vi "initializer.vi"(4 "Break":refnum<vi>) -> (0 "Cancelled?":bool, 2 "Dataflow Out":errorcluster)   [LabVIEW 2019]
panel:
  out "Button Cluster":T1
  out "Load Button Cluster":T2
  out "File Cluster":T3
  in  "Cancel Button":bool
  out "Endtime":dbl
  out "Starttime":dbl
  in  "Load Simulation File":bool
  out "Sim File Loaded":bool
  in  "LUA Simulation File":path
  out "Spec File Loaded":bool
  in  "Save Specs":bool
  out "Vali File Loaded":bool
  in  "Load Spec File":bool
  in  "Load Vali File":bool
  in  "LUA Specification File":path
  in  "LUA Validation File":path
  in  "Validate":bool
  out "# Lines":i32
  in  "Refresh Button":bool
  in  "Parameters":string(tree)="_3"
  in  "Run":bool
  # "Biogas Initializer"
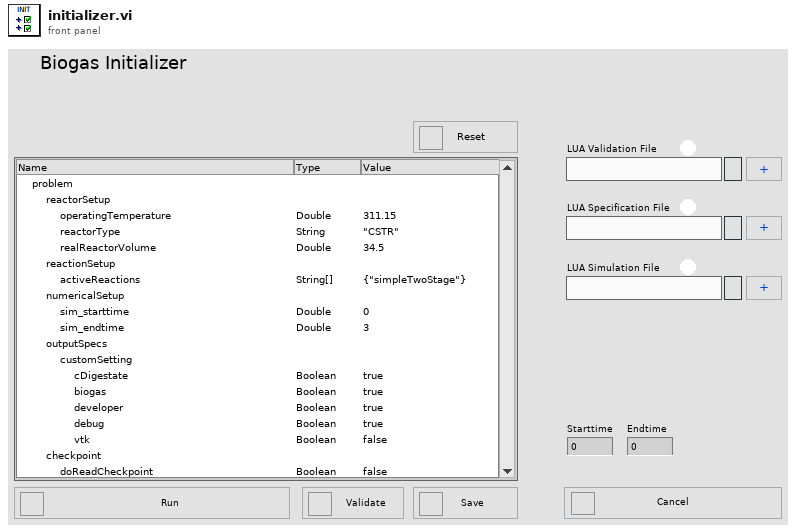
[diagram p1: front panel]
types:
  T1 = cluster{"Save Specs Button":refnum<vi>, "Cancel Button":refnum<vi>, "Run Button":refnum<vi>, "Refresh Button":refnum<vi>, "Validate Button":refnum<vi>}
  T2 = cluster{"Load Vali File":refnum<vi>, "Load Spec File":refnum<vi>, "Load Simulation File":refnum<vi>}
  T3 = cluster{"Sim File Loaded":refnum<vi>, "Vali File Loaded":refnum<vi>, "Spec File Loaded":refnum<vi>}
  T4 = cluster{"Vali File Loaded":refnum<vi>, "Spec File Loaded":refnum<vi>, "Sim File Loaded":refnum<vi>}
  T5 = typedef "LVPoint32TypeDef.ctl" = cluster{"Horizontal":i32, "Vertical":i32}
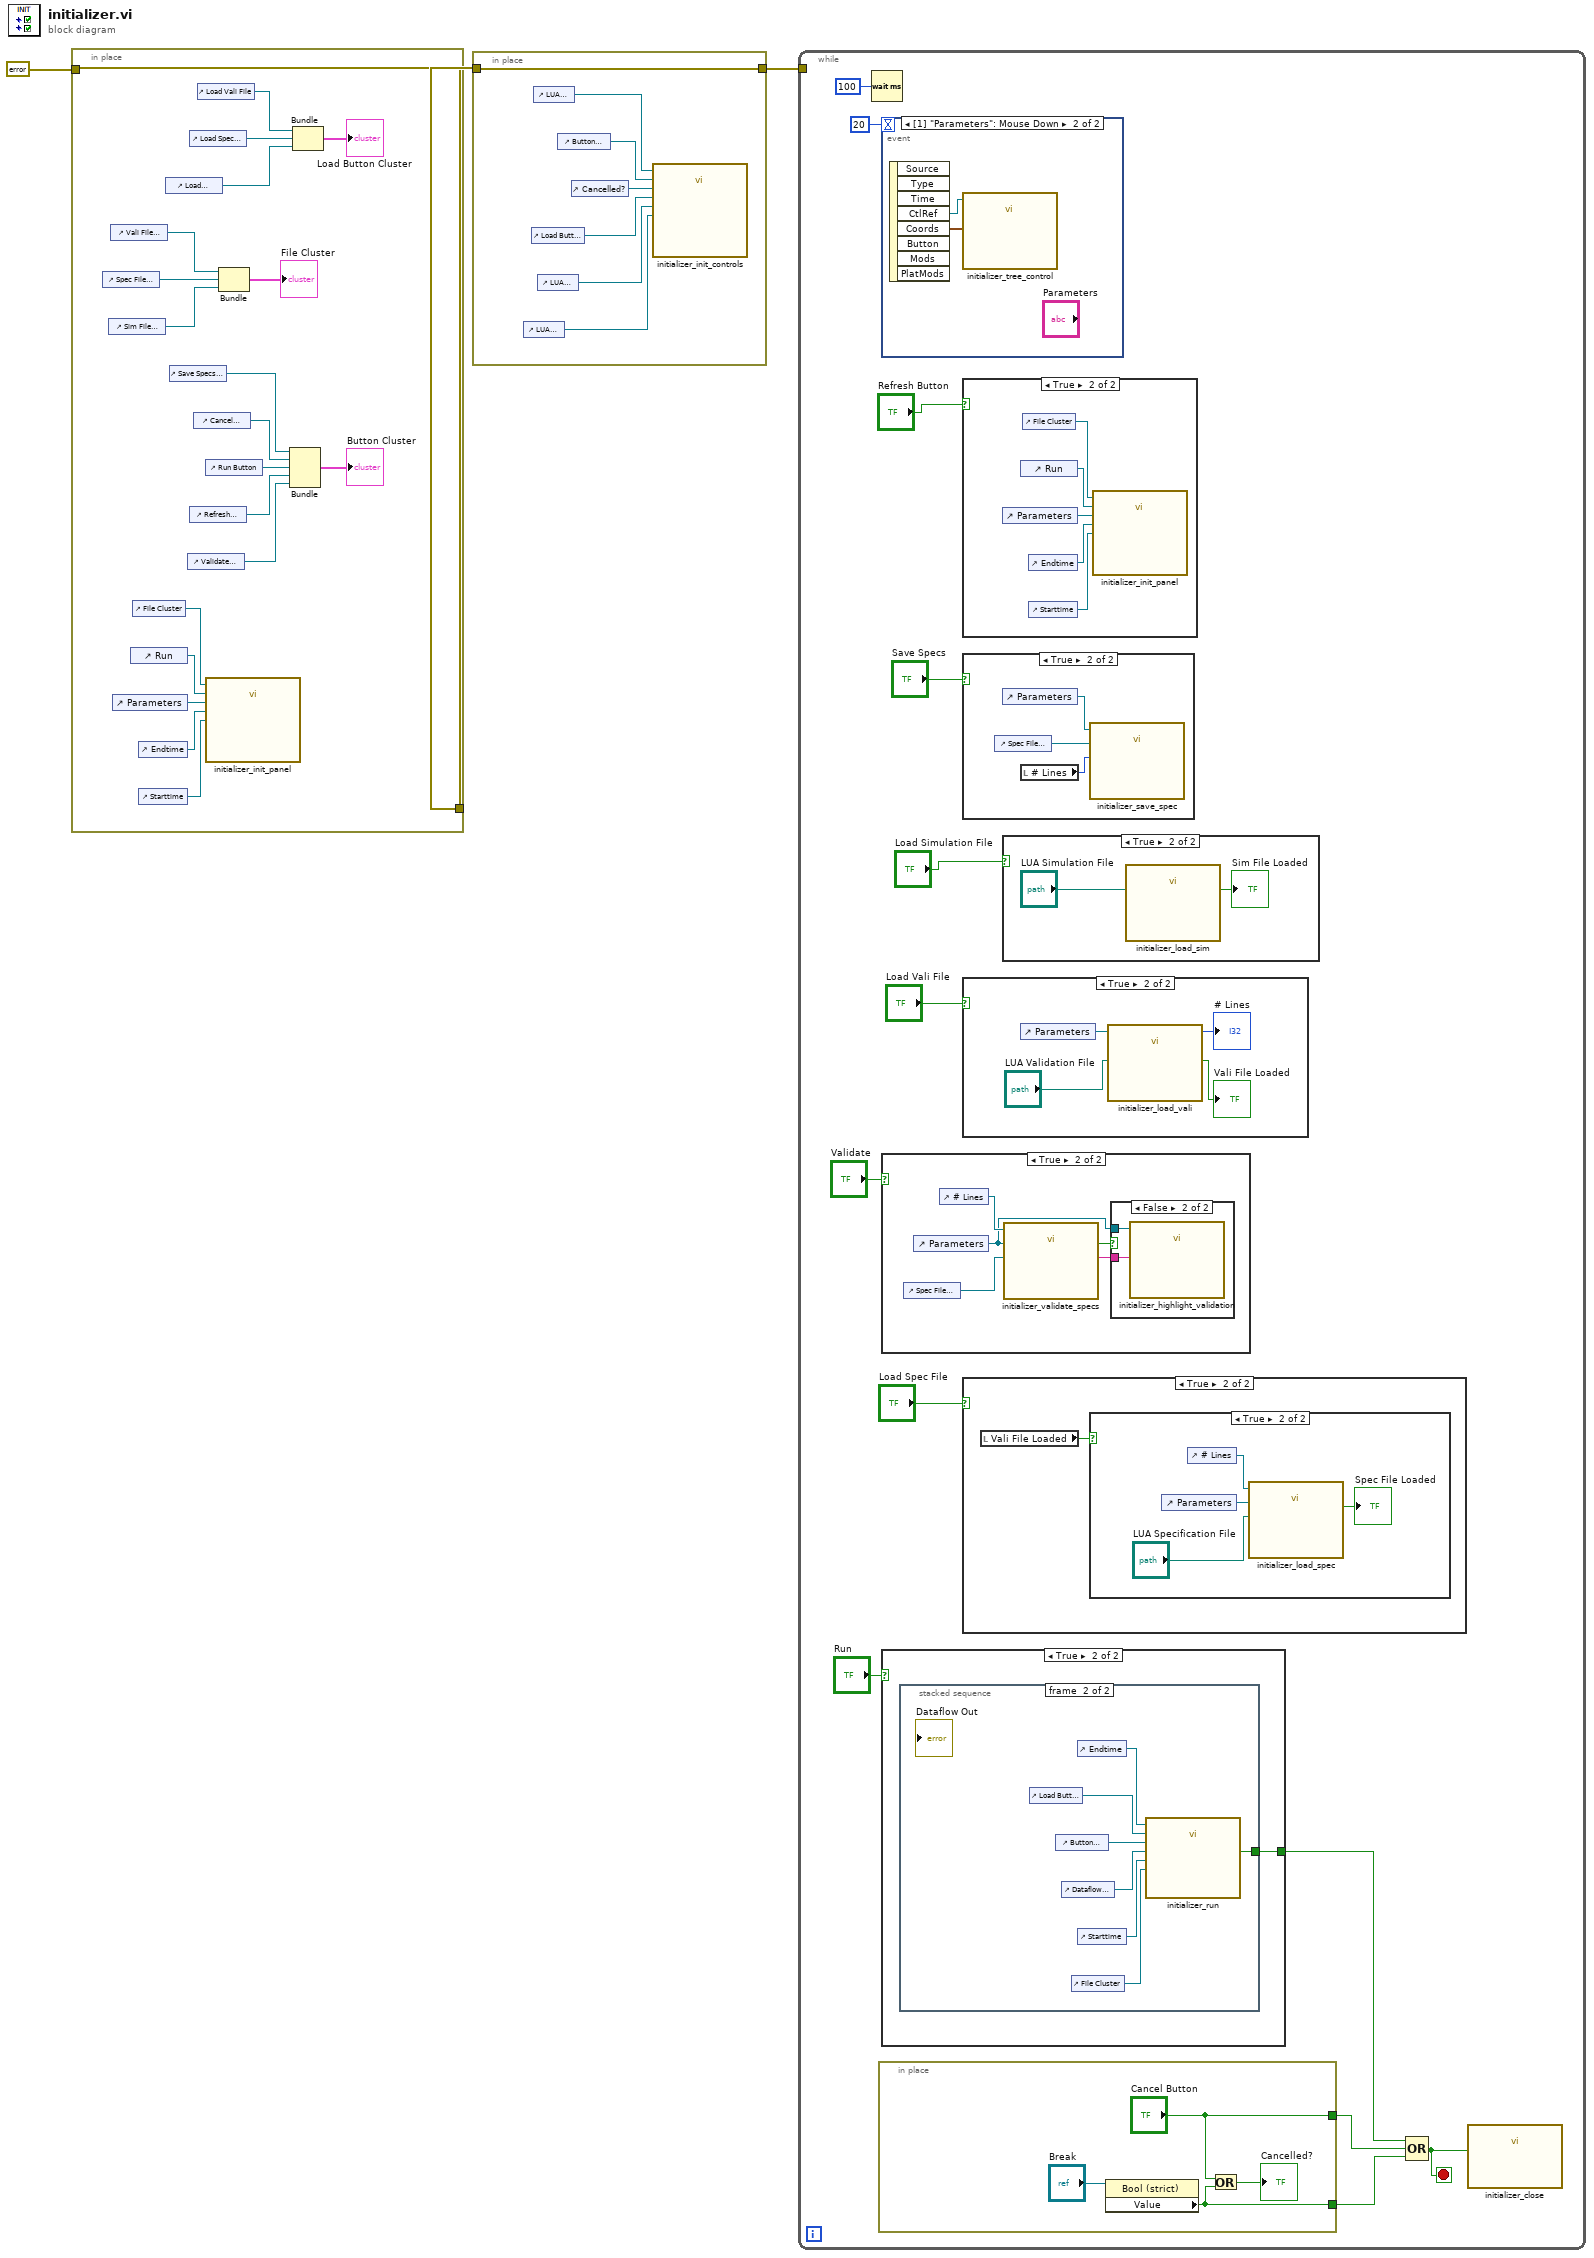
[diagram p0: block diagram]
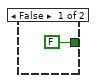
[diagram p2: hidden frame]
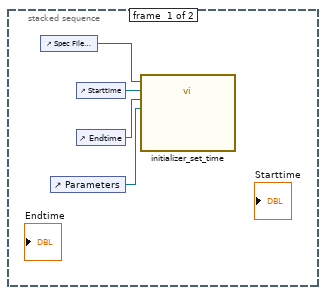
[diagram p3: hidden frame]
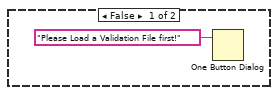
[diagram p9: hidden frame]
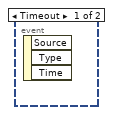
[diagram p11: hidden frame]
diagram:
  n1 = in-place {
    in-place-border: errorcluster {"status"=FALSE, "code"=0, "source"=""} ("error constant") -> [w19]
    in-place-border: [w19] -> w2
    n2 = control-ref of="Spec File Loaded"() -> (w11:refnum<vi>)
    n3 = control-ref of="Sim File Loaded"() -> (w12:refnum<vi>)
    n4 = control-ref of="Vali File Loaded"() -> (w10:refnum<vi>)
    n5 = control-ref of="Parameters"() -> (w23:refnum<vi>)
    n6 = control-ref of="Run"() -> (w20:refnum<vi>)
    n7 = control-ref of="File Cluster"() -> (w17:refnum<vi>)
    n8 = control-ref of="Endtime"() -> (w22:refnum<vi>)
    n9 = control-ref of="Starttime"() -> (w21:refnum<vi>)
    n10 = control-ref of="Load Simulation File"() -> (w14:refnum<vi>)
    n11 = control-ref of="Save Specs Button"() -> (w5:refnum<vi>)
    n12 = control-ref of="Validate Button"() -> (w9:refnum<vi>)
    n13 = control-ref of="Load Spec File"() -> (w15:refnum<vi>)
    n14 = control-ref of="Refresh Button"() -> (w8:refnum<vi>)
    n15 = control-ref of="Cancel Button"() -> (w6:refnum<vi>)
    n16 = control-ref of="Load Vali File"() -> (w16:refnum<vi>)
    n17 = control-ref of="Run Button"() -> (w7:refnum<vi>)
    n18 = call "initializer_init_panel.vi"("File Cluster"=w17, "Starttime"=w21, "Endtime"=w22, "Run Button"=w20, "Parameters Tree"=w23) -> ()  [unwired: 11 in]
    n19 = Bundle("Vali File Loaded"=w10, "Spec File Loaded"=w11, "Sim File Loaded"=w12) -> (→"File Cluster":T4)  [unwired: 1 in]
    n20 = Bundle("Save Specs Button"=w5, "Cancel Button"=w6, "Run Button"=w7, "Refresh Button"=w8, "Validate Button"=w9) -> (→"Button Cluster":T1)  [unwired: 1 in]
    n21 = Bundle("Load Vali File"=w16, "Load Spec File"=w15, "Load Simulation File"=w14) -> (→"Load Button Cluster":T2)  [unwired: 1 in]
  }
  n22 = in-place {
    in-place-border: [w30] -> w1
    in-place-border: w2 -> [w30]
    n23 = control-ref of="LUA Specification File"() -> (w27:refnum<vi>)
    n24 = control-ref of="Load Button Cluster"() -> (w25:refnum<vi>)
    n25 = control-ref of="LUA Simulation File"() -> (w28:refnum<vi>)
    n26 = control-ref of="LUA Validation File"() -> (w26:refnum<vi>)
    n27 = control-ref of="Button Cluster"() -> (w24:refnum<vi>)
    n28 = control-ref of="Cancelled?"() -> (w29:refnum<vi>)
    n29 = call "initializer_init_controls.vi"("LUA Simulation File"=w28, "Button Cluster"=w24, "Cancelled?"=w29, "Load Button Cluster"=w25, "LUA Specification File"=w27, "LUA Validation File"=w26) -> ()  [unwired: 14 in]
  }
  n30 = while {
    tunnel: w1 -> [_]
    stop <- w33 stop-if-true
    n31 = Wait (ms)(milliseconds to wait=u32 100) -> ()  [unwired: 1 out]
    n32 = in-place {
      in-place-border: ["Cancel Button"] -> w32
      in-place-border: [w44] -> w31
      n33 = property class="Bool (strict)"(reference="Break") -> ("Value"=w44:bool)  [unwired: 1 in, 2 out]
      n34 = Or(x="Cancel Button", y=w44) -> (x .or. y?=→"Cancelled?":bool)
    }
    n35 = event shown="[1] \"Parameters\": Mouse Down" {
      selector: _ -> [_ _]
      dyn-events: _ -> [_ _]
      timeout: 20 -> [_ _]
      event Timeout {
        n36 = event-data() -> ()  [unwired: 1 in, 3 out]
      }
      event "Parameters": Mouse Down {
        n37 = event-data() -> ("CtlRef"=w83:refnum<vi>, "Coords"=w84:T5)  [unwired: 1 in, 6 out]
        n38 = call "initializer_tree_control.vi"("Point"=w84, "Parameters Tree"=w83) -> ()  [unwired: 10 in]
      }
    }
    n39 = case shown="True" "Validate" {
      frame False {
      }
      frame True {
        n40 = control-ref of="Spec File Loaded"() -> (w67:refnum<vi>)
        n41 = control-ref of="Parameters"() -> (w68:refnum<vi>)
        n42 = control-ref of="# Lines"() -> (w70:refnum<vi>)
        n43 = call "initializer_validate_specs.vi"("Spec File Loaded?"=w67, "Parameters Tree"=w68, "# Lines"=w70) -> ("validationErrors"=w69:string, "Valid?"=w66:bool)  [unwired: 6 in, 1 out]
        n44 = case shown="False" w66 {
          tunnel: w69 -> [_ w72]
          tunnel: w68 -> [_ w71]
          frame True {
          }
          frame False {
            n45 = call "initializer_highlight_validation.vi"("validationErrors"=w72, "Parameters Tree"=w71) -> ()  [unwired: 10 in]
          }
        }
      }
    }
    n46 = case shown="True" "Run" {
      tunnel: [FALSE w49] -> w34
      frame False {
      }
      frame True {
        n47 = stacked-sequence {
          tunnel: [_ w60] -> w49
          frame #0 {
            n48 = control-ref of="Spec File Loaded"() -> (w51:refnum<vi>)
            n49 = control-ref of="Parameters"() -> (w50:refnum<vi>)
            n50 = control-ref of="Starttime"() -> (w53:refnum<vi>)
            n51 = control-ref of="Endtime"() -> (w52:refnum<vi>)
            n52 = call "initializer_set_time.vi"("Parameters Tree"=w50, "Endtime"=w52, "Starttime"=w53, "Spec File Loaded?"=w51) -> ()  [unwired: 8 in]
          }
          frame #1 {
            n53 = control-ref of="Load Button Cluster"() -> (w55:refnum<vi>)
            n54 = control-ref of="Button Cluster"() -> (w54:refnum<vi>)
            n55 = control-ref of="Dataflow Out"() -> (w59:refnum<vi>)
            n56 = control-ref of="File Cluster"() -> (w56:refnum<vi>)
            n57 = control-ref of="Endtime"() -> (w57:refnum<vi>)
            n58 = control-ref of="Starttime"() -> (w58:refnum<vi>)
            n59 = call "initializer_run.vi"("Endtime"=w57, "Load Button Cluster"=w55, "Button Cluster"=w54, "Dataflow Out"=w59, "File Cluster"=w56, "Starttime"=w58) -> ("Checkbox"=w60:bool)  [unwired: 21 in]
          }
        }
      }
    }
    n60 = case shown="True" "Refresh Button" {
      frame False {
      }
      frame True {
        n61 = control-ref of="Parameters"() -> (w89:refnum<vi>)
        n62 = control-ref of="Run"() -> (w86:refnum<vi>)
        n63 = control-ref of="File Cluster"() -> (w85:refnum<vi>)
        n64 = control-ref of="Endtime"() -> (w87:refnum<vi>)
        n65 = control-ref of="Starttime"() -> (w88:refnum<vi>)
        n66 = call "initializer_init_panel.vi"("File Cluster"=w85, "Starttime"=w88, "Endtime"=w87, "Run Button"=w86, "Parameters Tree"=w89) -> ()  [unwired: 11 in]
      }
    }
    n67 = case shown="True" "Save Specs" {
      frame False {
      }
      frame True {
        n68 = control-ref of="Spec File Loaded"() -> (w63:refnum<vi>)
        n69 = control-ref of="Parameters"() -> (w64:refnum<vi>)
        n70 = local read "# Lines"() -> (w65:i32)
        n71 = call "initializer_save_spec.vi"("# Lines"=w65, "Spec File Loaded?"=w63, "Parameters Tree"=w64) -> ()  [unwired: 9 in]
      }
    }
    n72 = case shown="True" "Load Vali File" {
      frame False {
      }
      frame True {
        n73 = control-ref of="Parameters"() -> (w81:refnum<vi>)
        n74 = call "initializer_load_vali.vi"("LUA Validation File"="LUA Validation File", "Parameters Tree"=w81) -> ("Vali File Loaded"=→"Vali File Loaded":bool, "# Lines"=→"# Lines":i32)  [unwired: 8 in]
      }
    }
    n75 = case shown="True" "Load Spec File" {
      frame False {
      }
      frame True {
        n76 = local read "Vali File Loaded"() -> (w73:bool)
        n77 = case shown="True" w73 {
          frame False {
            n78 = One Button Dialog(message="Please Load a Validation File first!") -> ()  [unwired: 1 in, 1 out]
          }
          frame True {
            n79 = control-ref of="Parameters"() -> (w77:refnum<vi>)
            n80 = control-ref of="# Lines"() -> (w78:refnum<vi>)
            n81 = call "initializer_load_spec.vi"("LUA Specification File"="LUA Specification File", "Parameters Tree"=w77, "# Lines"=w78) -> ("Spec File Loaded"=→"Spec File Loaded":bool)  [unwired: 8 in]
          }
        }
      }
    }
    n82 = case shown="True" "Load Simulation File" {
      frame False {
      }
      frame True {
        n83 = call "initializer_load_sim.vi"("LUA Simulation File"="LUA Simulation File") -> ("Sim File Loaded"=→"Sim File Loaded":bool)  [unwired: 10 in]
      }
    }
    n84 = Compound Arithmetic op=OR(w34, w32, w31) -> (w33:bool)
    n85 = call "initializer_close.vi"("Close?"=w33) -> ()  [unwired: 11 in]
  }
